vi "Shooter Control Mode Converter.vi"(11 "Shooter Mode":T2(ring)) -> (3 "Internal Control Mode":T1(ring))   [LabVIEW 2011]
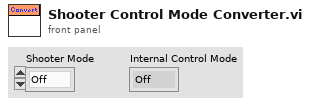
[diagram p1: front panel]
types:
  T1 = enum16{"Off", "Open Loop Control", "Closed Loop", "Top Spin", "Wait for Spindown"}
  T2 = enum16{"Off", "Open Loop Control", "Closed Loop Control", "Top Spin"}
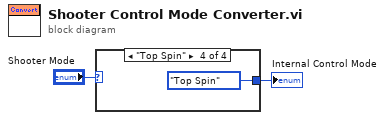
[diagram p0: block diagram]
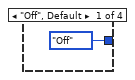
[diagram p2: hidden frame]
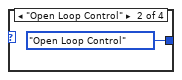
[diagram p3: hidden frame]
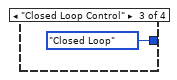
[diagram p4: hidden frame]
diagram:
  n1 = case shown="\"Top Spin\"" "Shooter Mode" {
    tunnel: [T1."Off" ("t") T1."Open Loop Control" ("t") T1."Closed Loop" ("t") T1."Top Spin" ("t")] -> w1
    frame "Off", Default {
    }
    frame "Open Loop Control" {
    }
    frame "Closed Loop Control" {
    }
    frame "Top Spin" {
    }
  }
  "Internal Control Mode" <- w1
